vi "Read Network Master.vi"(8 "error in (no error)":errorcluster, 11 "SMSD in":refnum<class "SMSD.lvclass">) -> (0 "error out":errorcluster, 2 "TCP Master":refnum<class "SMSD Master.lvclass">, 3 "SMSD out":refnum<class "SMSD.lvclass">)   [LabVIEW 2021, in "SMSD.lvclass"]
uses:
  SMSD.lvclass
  D:/my_projects/projects/Algorithms/Labview/21/Master CR/Master CR.lvclass
  Network Protocol/SMSD Master/SMSD Master.lvclass
  Master CR.lvclass/Master CR.ctl
  SMSD.lvclass/SMSD.ctl
  Master CR.lvclass
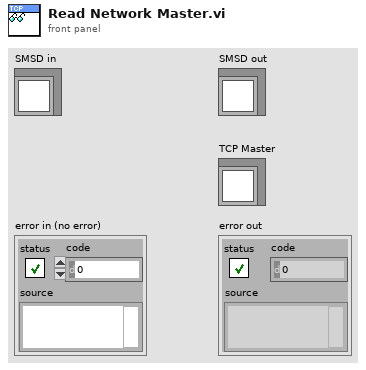
[diagram p1: front panel]
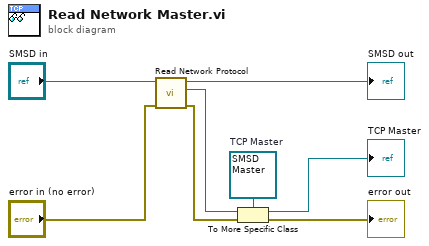
[diagram p0: block diagram]
diagram:
  w5 = refnum<class "SMSD Master.lvclass"> refnum  # TCP Master
  n1 = call "Read Network Protocol.vi"("error in (no error)"="error in (no error)", "Master CR in"="SMSD in") -> ("error out"=w3:errorcluster, "Network Protocol"=w4:refnum<class "Network Protocol.lvclass">, "Master CR out"=→"SMSD out":refnum<class "SMSD.lvclass">)  [unwired: 7 in]
  n2 = To More Specific Class(target class=w5, reference=w4, error in=w3) -> (specific class reference=→"TCP Master":refnum<class "SMSD Master.lvclass">, error out=→"error out":errorcluster)
